vi "isSearchGoalNode.vi"(8 "error in (no error)":errorcluster, 10 "PossibleSearchGoal in":refnum<data-value>, 11 "MultiTree in":refnum<class "MultiTree.lvclass">) -> (0 "error out":errorcluster, 1 "IsNode":bool, 2 "PossibleSearchGoal out":refnum<data-value>, 3 "MultiTree out":refnum<class "MultiTree.lvclass">)   [LabVIEW 2014, in "MultiTree.lvlib" / "MultiTree.lvclass"]
uses:
  <userlib>/AdvancedDataStructures/ClassBased/MultiTree/MultiTree.lvclass
  <userlib>/AdvancedDataStructures/ClassBased/MultiTreeNode/MultiTreeNode.lvclass
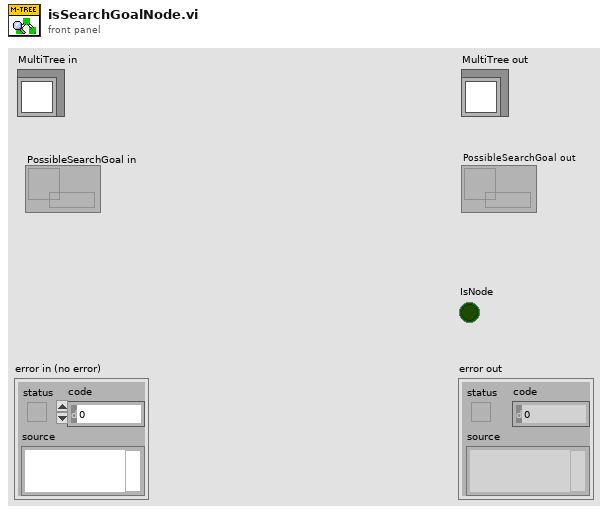
[diagram p1: front panel]
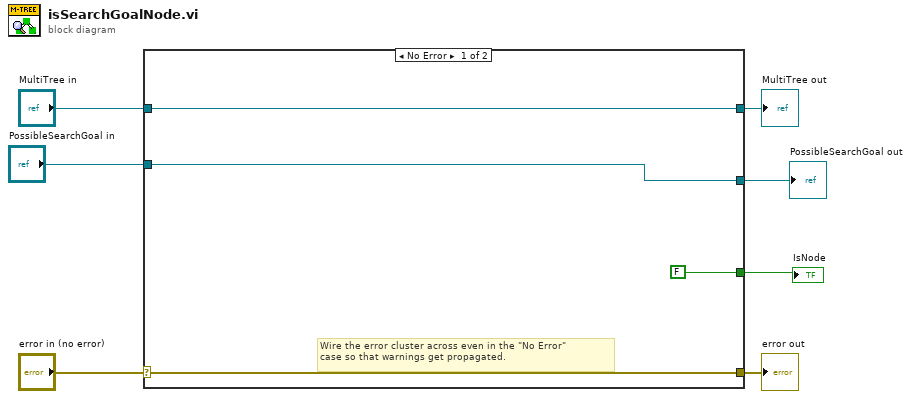
[diagram p0: block diagram]
diagram:
  n1 = case shown="No Error" "error in (no error)" {
    selector: "error in (no error)" -> [w10 w13]
    tunnel: [w10 w13] -> w6
    tunnel: [w11 w12] -> w4
    tunnel: "MultiTree in" -> [w11 w12]
    tunnel: [FALSE _] -> w3
    tunnel: [w8 _] -> w2
    tunnel: "PossibleSearchGoal in" -> [w8 _]
    frame No Error {
      # "Wire the error cluster across even in the \"No Error\"\ncase so that warnings get propagated."
    }
    frame Error {
    }
  }
  "error out" <- w6
  "MultiTree out" <- w4
  "PossibleSearchGoal out" <- w2
  "IsNode" <- w3
